vi "Example_MTMLoad1_ConstantCurrent.vi"() -> ()   [LabVIEW 2021, in "BrainStem2_LabVIEW_Library.lvlib"]
uses:
  BrainStem2_LabVIEW_Library.lvlib
panel:
  out "Output Current":i32
  out "Output Voltage":i32
  out "Device Serial Number":u32 format="%x"
  in  "Set Voltage Max Limit(uV)":i32
  in  "Set Current (uA)":i32
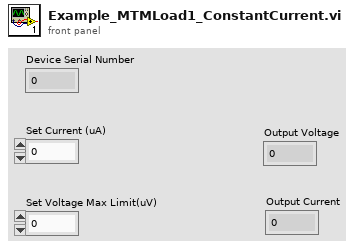
[diagram p1: front panel]
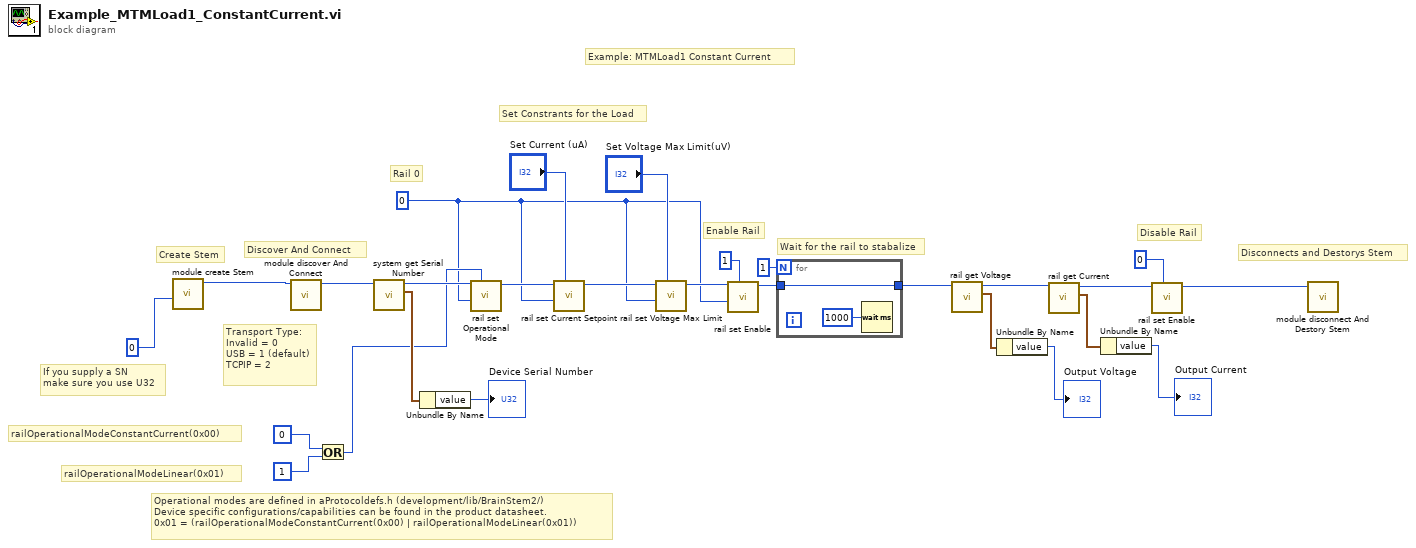
[diagram p0: block diagram]
diagram:
  w12 = u32 0
  # "Example: MTMLoad1 Constant Current"
  # "Set Constrants for the Load"
  # "railOperationalModeLinear(0x01)"
  # "railOperationalModeConstantCurrent(0x00)"
  # "Enable Rail"
  # "Disable Rail"
  # "Wait for the rail to stabalize"
  # "Rail 0"
  # "Operational modes are defined in aProtocoldefs.h (development/lib/BrainStem2/)\nDevice specific configurations/capabilities can be found in the product datasheet.\n0x01 = (railOperationalModeConstantCurrent(0x00) | railOperationalModeLinear(0x01))"
  # "Disconnects and Destorys Stem"
  # "Create Stem"
  # "Discover And Connect"
  # "If you supply a SN\nmake sure you use U32"
  # "Transport Type:\nInvalid = 0\nUSB = 1 (default)\nTCPIP = 2"
  n1 = call "module create Stem.vi"("sn"=u32 0) -> ("id out"=w27:u32)  [unwired: 8 in, 2 out]
  n2 = call "module discover And Connect.vi"("id"=w27) -> ("id out"=w25:u32)  [unwired: 8 in, 2 out]
  n3 = Or(x=u32 0, y=u32 1) -> (x .or. y?=w19:u32)
  n4 = call "system get Serial Number.vi"("id"=w25) -> ("result out"=w24:cluster{"value":i32, "error":i32}, "id out"=w20:u32)  [unwired: 8 in, 1 out]
  n5 = Unbundle By Name(w24) -> ("value"=→"Device Serial Number":i32)
  n6 = call "rail set Operational Mode.vi"("mode"=w19, "index"=w12, "id"=w20) -> ("id out"=w18:u32)  [unwired: 6 in, 2 out]
  n7 = call "rail set Current Setpoint.vi"("microamps"="Set Current (uA)", "index"=w12, "id"=w18) -> ("id out"=w15:u32)  [unwired: 6 in, 2 out]
  n8 = call "rail set Voltage Max Limit.vi"("microvolts"="Set Voltage Max Limit(uV)", "index"=w12, "id"=w15) -> ("id out"=w14:u32)  [unwired: 6 in, 2 out]
  n9 = call "rail set Enable.vi"("bEnable"=u32 1, "index"=w12, "id"=w14) -> ("id out"=w10:u32)  [unwired: 6 in, 2 out]
  n10 = for {
    N: 1 -> [_]
    tunnel: w10 -> [w28]
    tunnel: [w28] -> w9
    n11 = Wait (ms)(milliseconds to wait=u32 1000) -> ()  [unwired: 1 out]
  }
  n12 = call "rail get Voltage.vi"("id"=w9) -> ("result out"=w5:cluster{"value":i32, "error":i32}, "id out"=w8:u32)  [unwired: 8 in, 1 out]
  n13 = Unbundle By Name(w5) -> ("value"=→"Output Voltage":i32)
  n14 = call "rail get Current.vi"("id"=w8) -> ("result out"=w3:cluster{"value":i32, "error":i32}, "id out"=w7:u32)  [unwired: 8 in, 1 out]
  n15 = Unbundle By Name(w3) -> ("value"=→"Output Current":i32)
  n16 = call "rail set Enable.vi"("bEnable"=u32 0, "id"=w7) -> ("id out"=w1:u32)  [unwired: 7 in, 2 out]
  n17 = call "module disconnect And Destory Stem.vi"("id"=w1) -> ()  [unwired: 8 in, 3 out]
